vi "Julian_project5.vi"() -> ()   [LabVIEW 2020]
uses:
  enum_ctl.ctl
  <vilib>/Utility/file.llb/Read Delimited Spreadsheet (string).vi
  <vilib>/Utility/file.llb/Write Delimited Spreadsheet (string).vi
panel:
  out "?":string
  out "all 3 match":bool
  out "Incorrect":i32
  out "Waveform Graph 2":dbl[](graph)
  in  "simulation mode":bool
  in  "stop":bool
  out "Tab Control":enum32{"Login", "S.H.I.T", "Database"}(tab)
  in  "ID":string="Chad Davis"
  in  "Enter button":bool
  in  "Pin":string
  in  "Name":string="Chad Davis"
  in  "Logout":bool
  out "?":string
  out "Waveform Chart":dbl(graph)
  out "Waveform Graph":dbl[](graph)
  in  "Boolean":bool
  in  "Database":bool
  in  "Save Database":bool
  in  "all rows":string[][](array[string])
  in  "Logout 2":bool caption="Logout"
  in  "Retrieve Database":path
  # "All Data"
  # "Last 100"
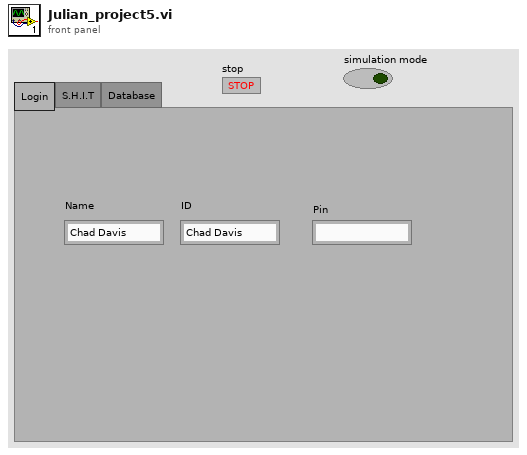
[diagram p1: front panel]
types:
  T1 = typedef "enum_ctl.ctl" = enum16{"Login", "S.H.I.T", "Database"}
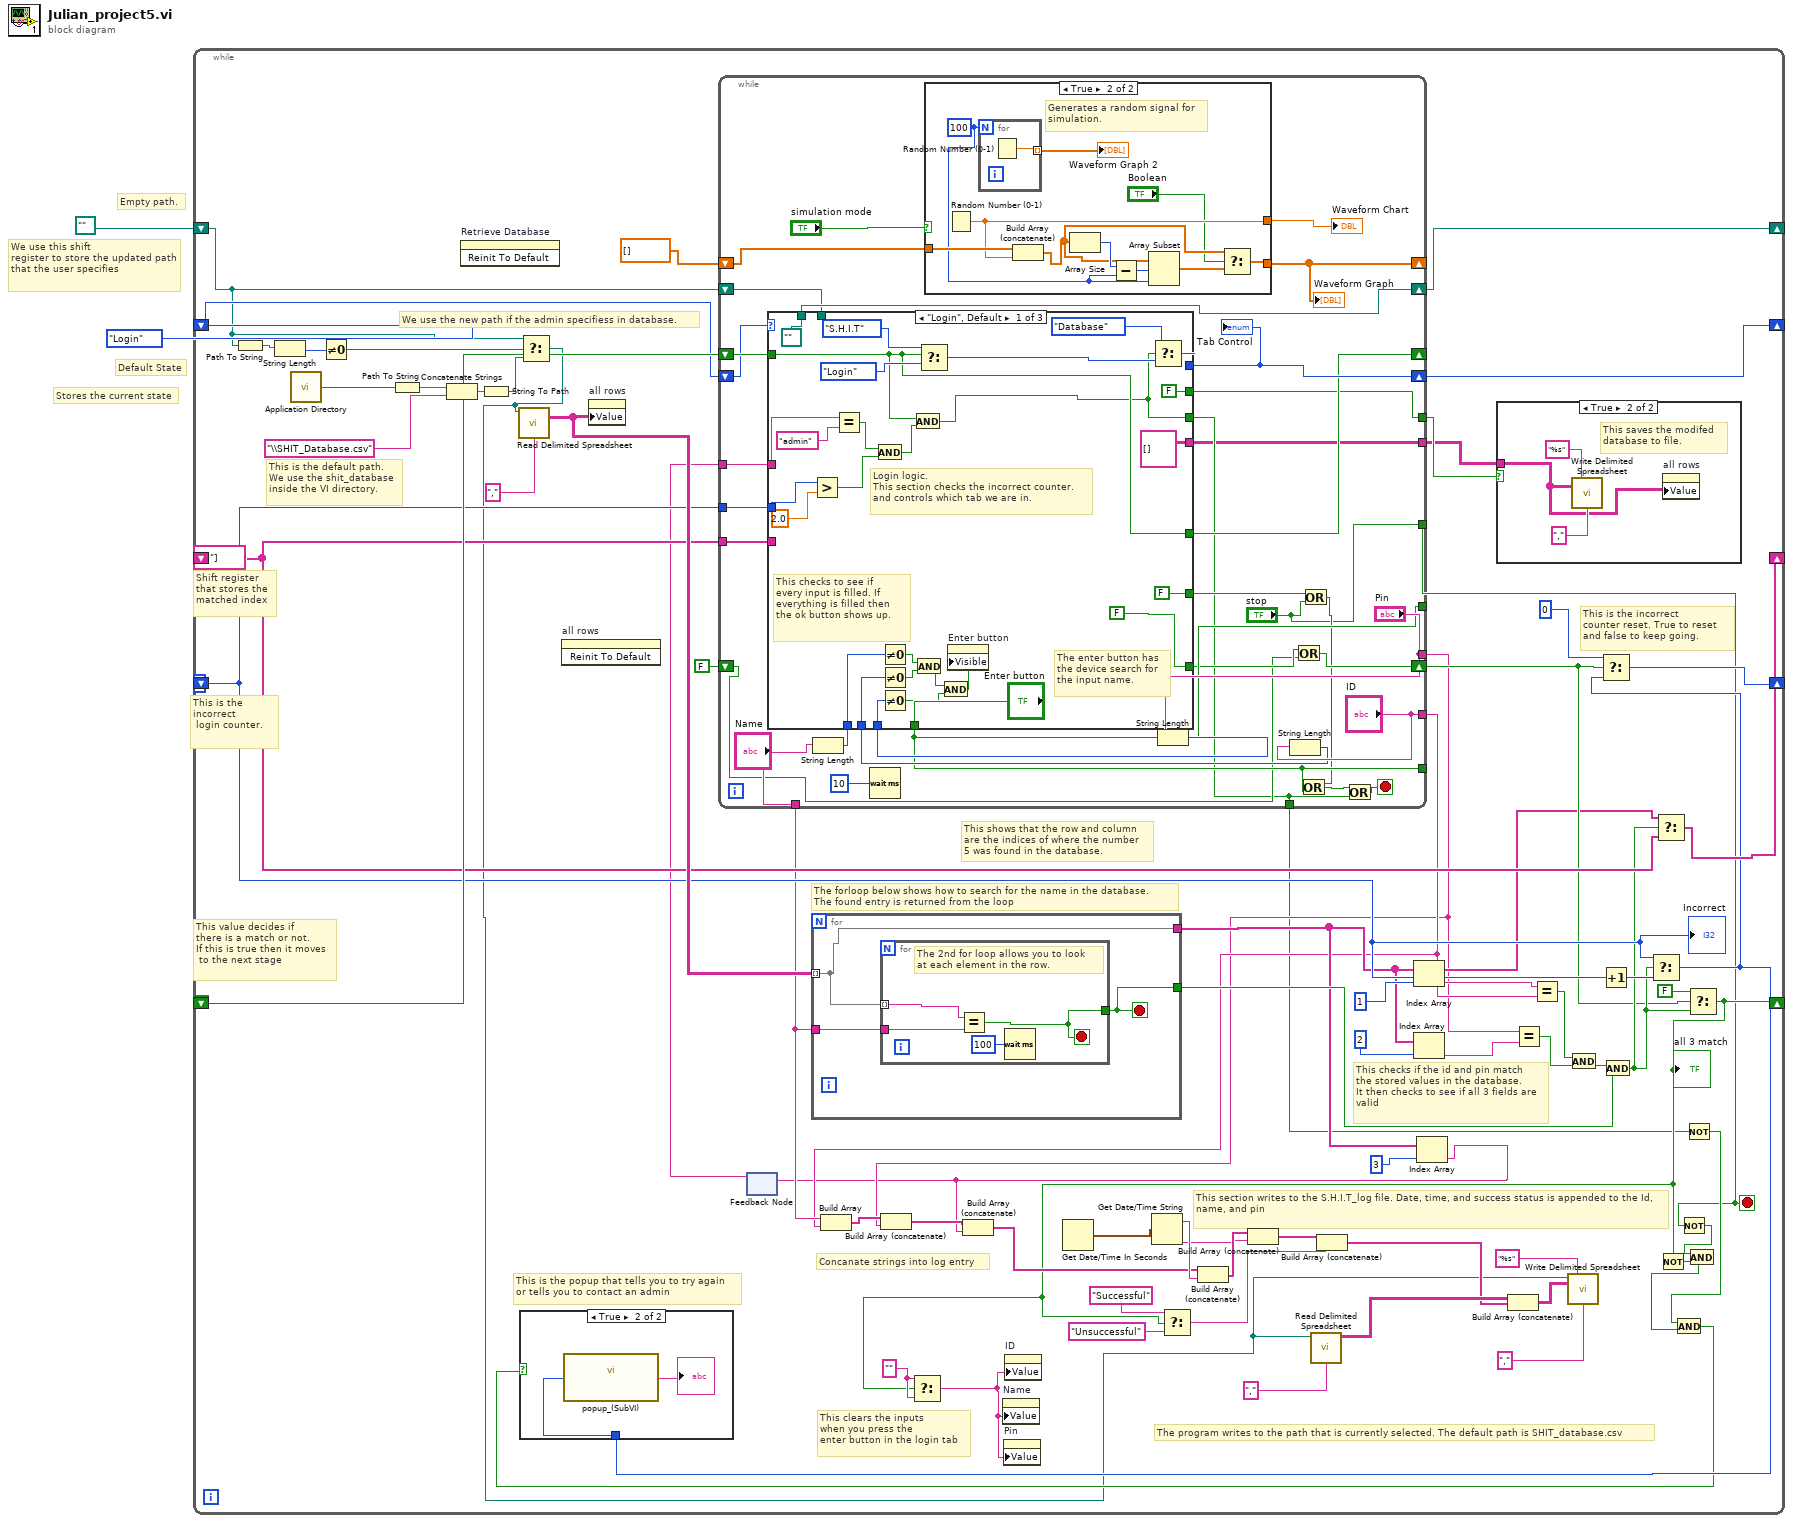
[diagram p0: block diagram]
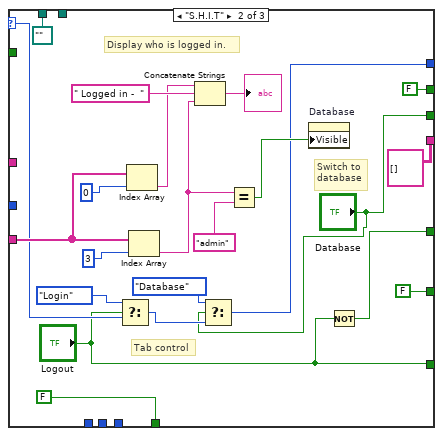
[diagram p4: hidden frame]
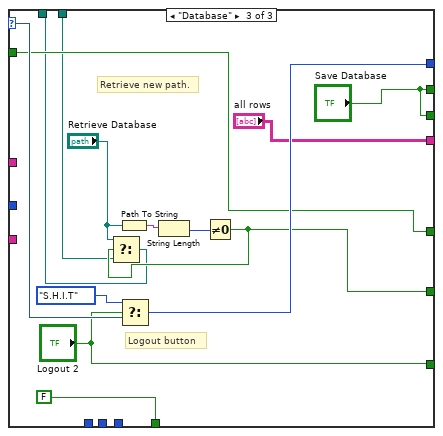
[diagram p5: hidden frame]
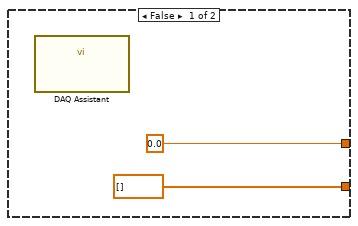
[diagram p6: hidden frame]
diagram:
  # "Stores the current state"
  # "We use this shift\nregister to store the updated path that the user specifies"
  # "Empty path."
  # "Default State"
  # "Shift register\nthat stores the\nmatched index"
  # "This is the incorrect\n login counter."
  # "This value decides if\nthere is a match or not.\nIf this is true then it moves\n to the next stage"
  n1 = while {
    shift-right: [w66] -> _
    shift-left: enum_ctl."Login" -> [w51]
    shift-right: [w16] -> _
    shift-left: FALSE -> [w62]
    shift-right: [w56] -> _
    shift-left: 0 -> [w59]
    shift-right: [w58] -> _
    shift-left: string[] ["0"] ("all rows") -> [w57]
    shift-right: [w28] -> _
    shift-left: path "" -> [w29]
    stop <- w10 stop-if-true
    w26 = ""
    # "We use the new path if the admin specifiess in database."
    # "Concanate strings into log entry"
    # "This is the default path. \nWe use the shit_database\ninside the VI directory."
    # "This is the incorrect\ncounter reset. True to reset and false to keep going."
    # "The program writes to the path that is currently selected. The default path is SHIT_database.csv"
    # "This section writes to the S.H.I.T_log file. Date, time, and success status is appended to the Id, name, and pin"
    # "This is the popup that tells you to try again\nor tells you to contact an admin"
    # "This clears the inputs\nwhen you press the \nenter button in the login tab"
    # "This checks if the id and pin match\nthe stored values in the database.\nIt then checks to see if all 3 fields are\nvalid"
    # "This shows that the row and column\nare the indices of where the number\n5 was found in the database."
    # "The forloop below shows how to search for the name in the database.\nThe found entry is returned from the loop"
    n2 = Path To String(path=w29) -> (string=w48:string)
    n3 = String Length(string=w48) -> (length=w47:i32)
    n4 = call <vilib>:"Application Directory.vi"() -> ("Application Directory"=w46:path)
    n5 = Not Equal To 0?(x=w47) -> (x != 0?=w44:bool)
    n6 = Path To String(path=w46) -> (string=w76:string)
    n7 = Concatenate Strings(w76, "\\SHIT_Database.csv" ("string")) -> (w74:string)
    n8 = invoke on="Retrieve Database" class="Path" method="Reinit To Default"() -> ()  [unwired: 3 in, 3 out]
    n9 = String To Path(string=w74) -> (path=w45:path)
    n10 = Select(t=w29, s=w44, f=w45) -> (s? t:f=w6:path)
    n11 = call-poly <vilib>:"Read Delimited Spreadsheet.vi"("file path (dialog if empty)"=w6, "delimiter (\\t)"="," ("delimiter (\\t)")) -> ("all rows"=w71:string[][])  [unwired: 8 in, 5 out]
    n12 = invoke on="all rows" class="Arr (strict)" method="Reinit To Default"() -> ()  [unwired: 3 in, 3 out]
    n13 = property on="all rows" class="Arr (strict)"("Value"=w71) -> ()  [unwired: 2 in, 2 out]
    n14 = feedback #1() -> (w50:string)  [unwired: 1 in]
    n15 = while {
      tunnel: [w105] -> _
      shift-right: [w117] -> _
      shift-left: dbl[] [] -> [w108]
      tunnel: ["Name"] -> w24
      tunnel: [w105] -> _
      tunnel: ["ID"] -> w23
      tunnel: ["Pin"] -> w21
      tunnel: w50 -> [w109]
      tunnel: w59 -> [w107]
      tunnel: ["stop"] -> w10
      tunnel: w57 -> [w104]
      shift-right: [w106] -> w66
      shift-left: w51 -> [w103]
      shift-right: [w102] -> w52
      shift-left: FALSE -> [w100]
      shift-right: [w99] -> _
      shift-left: w62 -> [w110]
      shift-right: [w96] -> w28
      shift-left: w29 -> [w94]
      tunnel: [w91] -> w14
      tunnel: [w89] -> w9
      tunnel: [w90] -> w8
      stop <- w92 stop-if-true
      n16 = String Length(string="Name") -> (length=w114:i32)
      n17 = Wait (ms)(milliseconds to wait=u32 10) -> ()  [unwired: 1 out]
      n18 = case shown="True" "simulation mode" {
        tunnel: [0.0 ("number: 0 to 1") w195] -> w119
        tunnel: w108 -> [_ w196]
        tunnel: [dbl[] [] w189] -> w117
        frame False {
          n19 = call "DAQ Assistant"() -> ()  [unwired: 12 in]
        }
        frame True {
          w192 = 100
          # "Generates a random signal for\nsimulation."
          n20 = Random Number (0-1)() -> (number: 0 to 1=w195:dbl)
          n21 = for {
            N: w192 -> [_]
            tunnel: [w197] -> w194 mode=indexing
            n22 = Random Number (0-1)() -> (number: 0 to 1=w197:dbl)
          }
          "Waveform Graph 2" <- w194
          n23 = Build Array (concatenate)(w196, w195) -> (w190:dbl[])
          n24 = Array Size(array=w190) -> (size(s)=w193:i32)
          n25 = Subtract(x=w193, y=w192) -> (x-y=w191:i32)
          n26 = Array Subset(array=w190, index=w191, length=w192) -> (w188:dbl[])
          n27 = Select(t=w190, s="Boolean", f=w188) -> (s? t:f=w189:dbl[])
        }
      }
      "Waveform Chart" <- w119
      "Waveform Graph" <- w117
      n28 = String Length(string="Pin") -> (length=w111:i32)
      n29 = String Length(string="ID") -> (length=w112:i32)
      n30 = case shown="\"Login\", Default" w103 {
        selector: w103 -> [_ w162 w182]
        tunnel: [w133 w152 w180] -> w106
        tunnel: w114 -> [w148 _ _]
        tunnel: ["Enter button" FALSE ("Enter button") FALSE ("Enter button")] -> w105
        tunnel: w112 -> [w146 _ _]
        tunnel: w111 -> [w145 _ _]
        tunnel: w110 -> [w127 _ w179]
        tunnel: w109 -> [w139 _ _]
        tunnel: w107 -> [w136 _ _]
        tunnel: w104 -> [_ w166 _]
        tunnel: [FALSE ("Logout") "Logout" "Logout 2"] -> w101
        tunnel: [w127 w161 w179] -> w99
        tunnel: [FALSE FALSE w176] -> w97
        tunnel: [path "" ("Retrieve Database") path "" ("Retrieve Database") w173] -> w96
        tunnel: w94 -> [_ _ w175]
        tunnel: [w123 "Database" "Save Database"] -> w91
        tunnel: [string[][] [] ("all rows") string[][] [] ("all rows") "all rows"] -> w90
        tunnel: [FALSE ("Save Database") FALSE ("Save Database") "Save Database"] -> w89
        frame "Login", Default {
          # "Login logic.\nThis section checks the incorrect counter.\nand controls which tab we are in."
          # "The enter button has \nthe device search for \nthe input name."
          # "This checks to see if \nevery input is filled. If \neverything is filled then\nthe ok button shows up."
          n31 = Greater?(x=w136, y=2.0) -> (0:w135:bool)
          n32 = Equal?(x=w139, y="admin") -> (x = y?=w124:bool)
          n33 = And(x=w124, y=w135) -> (x .and. y?=w130:bool)
          n34 = Not Equal To 0?(x=w148) -> (x != 0?=w143:bool)
          n35 = Not Equal To 0?(x=w146) -> (x != 0?=w144:bool)
          n36 = Not Equal To 0?(x=w145) -> (x != 0?=w141:bool)
          n37 = And(x=w127, y=w130) -> (x .and. y?=w123:bool)
          n38 = And(x=w143, y=w144) -> (x .and. y?=w142:bool)
          n39 = Select(t=enum_ctl."S.H.I.T", s=w127, f=enum_ctl."Login") -> (s? t:f=w132:T1)
          n40 = And(x=w142, y=w141) -> (x .and. y?=w140:bool)
          n41 = property on="Enter button" class="Bool"("Visible"=w140) -> ()  [unwired: 2 in, 2 out]
          n42 = Select(t=enum_ctl."Database", s=w123, f=w132) -> (s? t:f=w133:T1)
        }
        frame "S.H.I.T" {
          # "Switch to\ndatabase"
          # "Tab control"
          # "Display who is logged in."
          n43 = Select(t=enum_ctl."Login", s="Logout", f=w162) -> (s? t:f=w154:T1)
          n44 = Index Array(array=w166, index=0) -> (element=w165:string)
          n45 = Index Array(array=w166, index=3) -> (element=w156:string)
          n46 = Concatenate Strings(w165, " Logged in -  " ("string"), w156) -> (→"?":string)
          n47 = Select(t=enum_ctl."Database", s="Database", f=w154) -> (s? t:f=w152:T1)
          n48 = Equal?(x=w156, y="admin" ("string")) -> (x = y?=w155:bool)
          n49 = property on="Database" class="Bool"("Visible"=w155) -> ()  [unwired: 2 in, 2 out]
          n50 = Not(x="Logout") -> (.not. x?=w161:bool)
        }
        frame "Database" {
          # "Logout button"
          # "Retrieve new path."
          n51 = Path To String(path="Retrieve Database") -> (string=w178:string)
          n52 = Select(t=enum_ctl."S.H.I.T", s="Logout 2", f=w182) -> (s? t:f=w180:T1)
          n53 = String Length(string=w178) -> (length=w177:i32)
          n54 = Not Equal To 0?(x=w177) -> (x != 0?=w176:bool)
          n55 = Select(t="Retrieve Database", s=w176, f=w175) -> (s? t:f=w173:path)
        }
      }
      "Tab Control" <- w106
      n56 = Or(x=w101, y=w100) -> (x .or. y?=w102:bool)
      n57 = Or(x=w97, y="stop") -> (x .or. y?=w98:bool)
      n58 = Or(x=w98, y=w105) -> (x .or. y?=w93:bool)
      n59 = Or(x=w93, y=w91) -> (x .or. y?=w92:bool)
    }
    n60 = for {
      tunnel: w71 -> [w83] mode=indexing
      tunnel: w24 -> [w84]
      tunnel: [w83] -> w25
      tunnel: [w82] -> w63
      stop <- w82 stop-if-true
      n61 = for {
        tunnel: w83 -> [w88] mode=indexing
        tunnel: [w85] -> w82
        tunnel: w84 -> [w86]
        stop <- w85 stop-if-true
        # "The 2nd for loop allows you to look\nat each element in the row."
        n62 = Equal?(x=w88, y=w86) -> (x = y?=w85:bool)
        n63 = Wait (ms)(milliseconds to wait=u32 100) -> ()  [unwired: 1 out]
      }
    }
    n64 = Build Array(w24, w23) -> (w22:string[])
    n65 = Build Array (concatenate)(w22, w21) -> (w20:string[])
    n66 = Get Date/Time In Seconds() -> (seconds since 1Jan1904=w39:timestamp)
    n67 = Get Date/Time String(seconds (now)=w39) -> (date string=w38:string, time string=w35:string)  [unwired: 2 in]
    n68 = call-poly <vilib>:"Read Delimited Spreadsheet.vi"("file path (dialog if empty)"=w6, "delimiter (\\t)"="," ("delimiter (\\t)")) -> ("all rows"=w40:string[][])  [unwired: 8 in, 5 out]
    n69 = Index Array(array=w25, index=1) -> (element=w69:string)
    n70 = Index Array(array=w25, index=2) -> (element=w67:string)
    n71 = Index Array(array=w25, index=3) -> (element=w19:string)
    n72 = feedback-in #1(w19) -> ()
    n73 = Build Array (concatenate)(w20, w19) -> (w18:string[])
    n74 = Build Array (concatenate)(w18, w38) -> (w36:string[])
    n75 = Build Array (concatenate)(w36, w35) -> (w34:string[])
    n76 = case shown="True" w9 {
      tunnel: w8 -> [_ w77]
      frame False {
      }
      frame True {
        # "This saves the modifed \ndatabase to file."
        n77 = call-poly <vilib>:"Write Delimited Spreadsheet.vi"("format (%s)"="%s" ("format (%.3f)"), "2D data"=w77, "delimiter (\\t)"="," ("delimiter (\\t)")) -> ()  [unwired: 11 in, 2 out]
        n78 = property on="all rows" class="Arr (strict)"("Value"=w77) -> ()  [unwired: 2 in, 2 out]
      }
    }
    n79 = Equal?(x=w21, y=w67) -> (x = y?=w64:bool)
    n80 = Equal?(x=w69, y=w23) -> (x = y?=w65:bool)
    n81 = And(x=w65, y=w64) -> ()  [unwired: 1 out]
    n82 = Increment(x=w59) -> (x+1=w60:i32)
    n83 = And(x=w64, y=w63) -> (x .and. y?=w54:bool)
    n84 = Select(t=w59, s=w54, f=w60) -> (s? t:f=w27:i32)
    n85 = Select(t=0, s=w52, f=w27) -> (s? t:f=w56:i32)
    n86 = Select(t=w25, s=w54, f=w57) -> (s? t:f=w58:string[])
    n87 = Not(x=w10) -> (.not. x?=w17:bool)
    n88 = Not(x=w14) -> (.not. x?=w11:bool)
    n89 = Select(t=FALSE, s=w52, f=w54) -> (s? t:f=w16:bool)
    "all 3 match" <- w16
    n90 = Select(t=w26, s=w16, f=w26) -> (s? t:f=w7:string)
    n91 = property on="Name" class="Str"("Value"=w7) -> ()  [unwired: 2 in, 2 out]
    n92 = property on="Pin" class="Str"("Value"=w7) -> ()  [unwired: 2 in, 2 out]
    n93 = property on="ID" class="Str"("Value"=w7) -> ()  [unwired: 2 in, 2 out]
    n94 = Select(t="Successful", s=w16, f="Unsuccessful" ("t")) -> (s? t:f=w30:string)
    n95 = Build Array (concatenate)(w34, w30) -> (w33:string[])
    n96 = Build Array (concatenate)(w40, w33) -> (w37:string[][])
    n97 = call-poly <vilib>:"Write Delimited Spreadsheet.vi"("file path (dialog if empty)"=w6, "format (%s)"="%s" ("format (%.3f)"), "2D data"=w37, "delimiter (\\t)"="," ("delimiter (\\t)")) -> ()  [unwired: 10 in, 2 out]
    n98 = Not(x=w16) -> (.not. x?=w15:bool)
    n99 = And(x=w17, y=w15) -> (x .and. y?=w12:bool)
    n100 = And(x=w11, y=w12) -> (x .and. y?=w13:bool)
    n101 = case shown="True" w13 {
      tunnel: w27 -> [_ w80]
      frame False {
      }
      frame True {
        n102 = call "popup_(SubVI).vi"("X"=w80) -> (3:→"?":string)  [unwired: 10 in]
      }
    }
    "Incorrect" <- w59
  }
